vi "serialization tests.vi"() -> ()   [LabVIEW 2013, in "EthernetIP tests.lvlib"]
uses:
  EthernetIP tests.lvlib
  configuration/EthernetIP configuration.lvclass
panel:
  out "modules equal":bool
  out "channels equal":bool
  out "no error":errorcluster
  out "no error":errorcluster
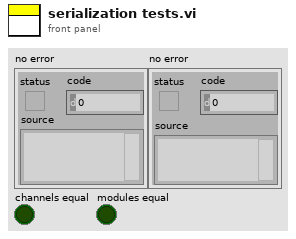
[diagram p1: front panel]
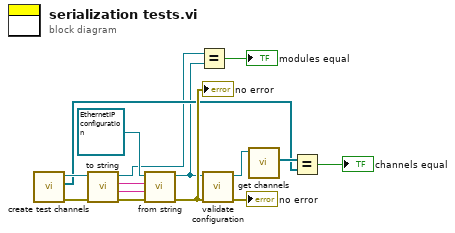
[diagram p0: block diagram]
diagram:
  n1 = call "create test channels.vi"() -> ("error out"=w8:errorcluster, "Array"=w5:refnum<class "EthernetIP Channel.lvclass">[], "EthernetIP configuration out"=w9:refnum<class "EthernetIP configuration.lvclass">)  [unwired: 7 in, 2 out]
  n2 = call-dynamic "to string.vi"("error in"=w8, "EthernetIP configuration in"=w9) -> ("error out"=w15:errorcluster, "data"=w14:string, "version"=w13:string, "EthernetIP configuration out"=w2:refnum<class "EthernetIP configuration.lvclass">)  [unwired: 6 in]
  n3 = call-dynamic "from string.vi"("error in"=w15, "data"=w14, "version"=w13, "EthernetIP configuration in"=refnum<class "EthernetIP configuration.lvclass"> refnum ("EthernetIP configuration")) -> ("error out"=w11:errorcluster, "EthernetIP configuration out"=w3:refnum<class "EthernetIP configuration.lvclass">)  [unwired: 6 in]
  "no error" <- w11
  n4 = Equal?(x=w2, y=w3) -> (x = y?=→"modules equal":bool)
  n5 = call-dynamic "validate configuration.vi"("error in"=w11, "EthernetIP configuration in"=w3) -> ("error out"=→"no error":errorcluster, "EthernetIP configuration out"=w7:refnum<class "EthernetIP configuration.lvclass">)  [unwired: 8 in]
  n6 = call-dynamic "get channels.vi"("EthernetIP configuration in"=w7) -> ("channels"=w6:refnum<class "TBM channel.lvclass">[])  [unwired: 9 in, 1 out]
  n7 = Equal?(x=w6, y=w5) -> (x = y?=→"channels equal":bool)
